vi "Control_giro_v4.vi"() -> ()   [LabVIEW 2025]
uses:
  <vilib>/addons/control/pid/pid.llb/PID (DBL).vi
  <vilib>/addons/control/pid/NI_PID_pid.lvlib
panel:
  in  "Boolean 2":bool
  in  "Boolean":bool
  out "valor_actual_ajustado":dbl
  out "setpoint_ajustado":dbl
  out "PWM":dynamicdata(graph) caption="Square"
  out "Señal B":i16(graph)
  out "Señal A":i16(graph)
  out "output":dbl format="%.2f"
  in  "PID gains":T1={"proportional gain (Kc)"=1.0, "integral time (Ti, min)"=0.01, "derivative time (Td, min)"=0.0} {"derivative time (Td, min)" format="%.3f"; "integral time (Ti, min)" format="%.3f"; "proportional gain (Kc)" format="%.3f"}
  out "Error (°)":dbl
  out "Sensor":dbl(knob) scale=0.0..359.0
  in  "SetPoint":dbl(knob) max=359.0 scale=0.0..359.0
  out "Posición (°)":dbl
  in  "Reestablecer cero":bool
  out "Pulsos":dbl
  in  "stop":bool
  # "ENCODER"
  # "SALIDA"
  # "PID"
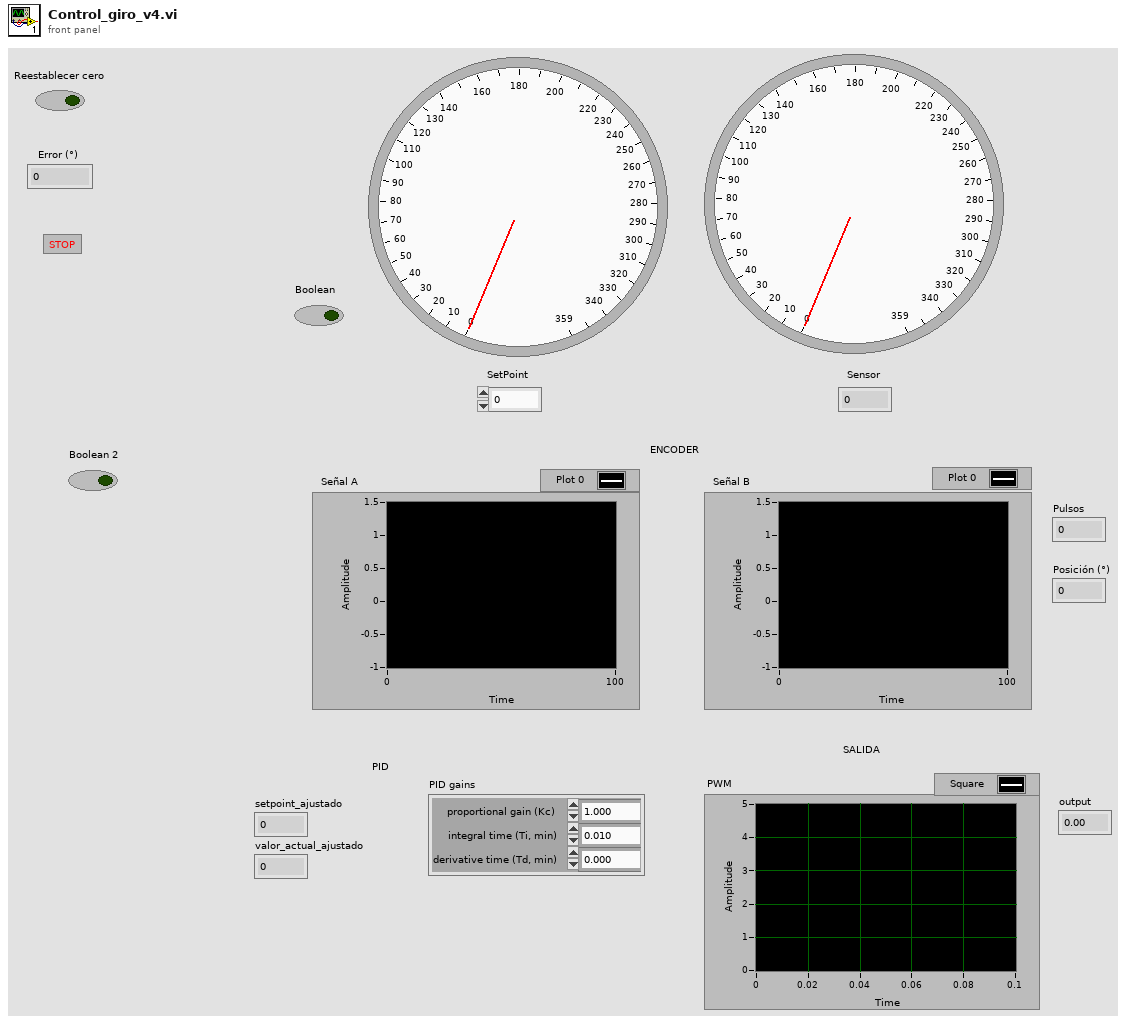
[diagram p1: front panel]
types:
  T1 = cluster{"proportional gain (Kc)":dbl, "integral time (Ti, min)":dbl, "derivative time (Td, min)":dbl}
  T2 = enum16{"Ini", "H1", "H2", "H3", "RES", "A1", "A2", "A3", "SUM"}
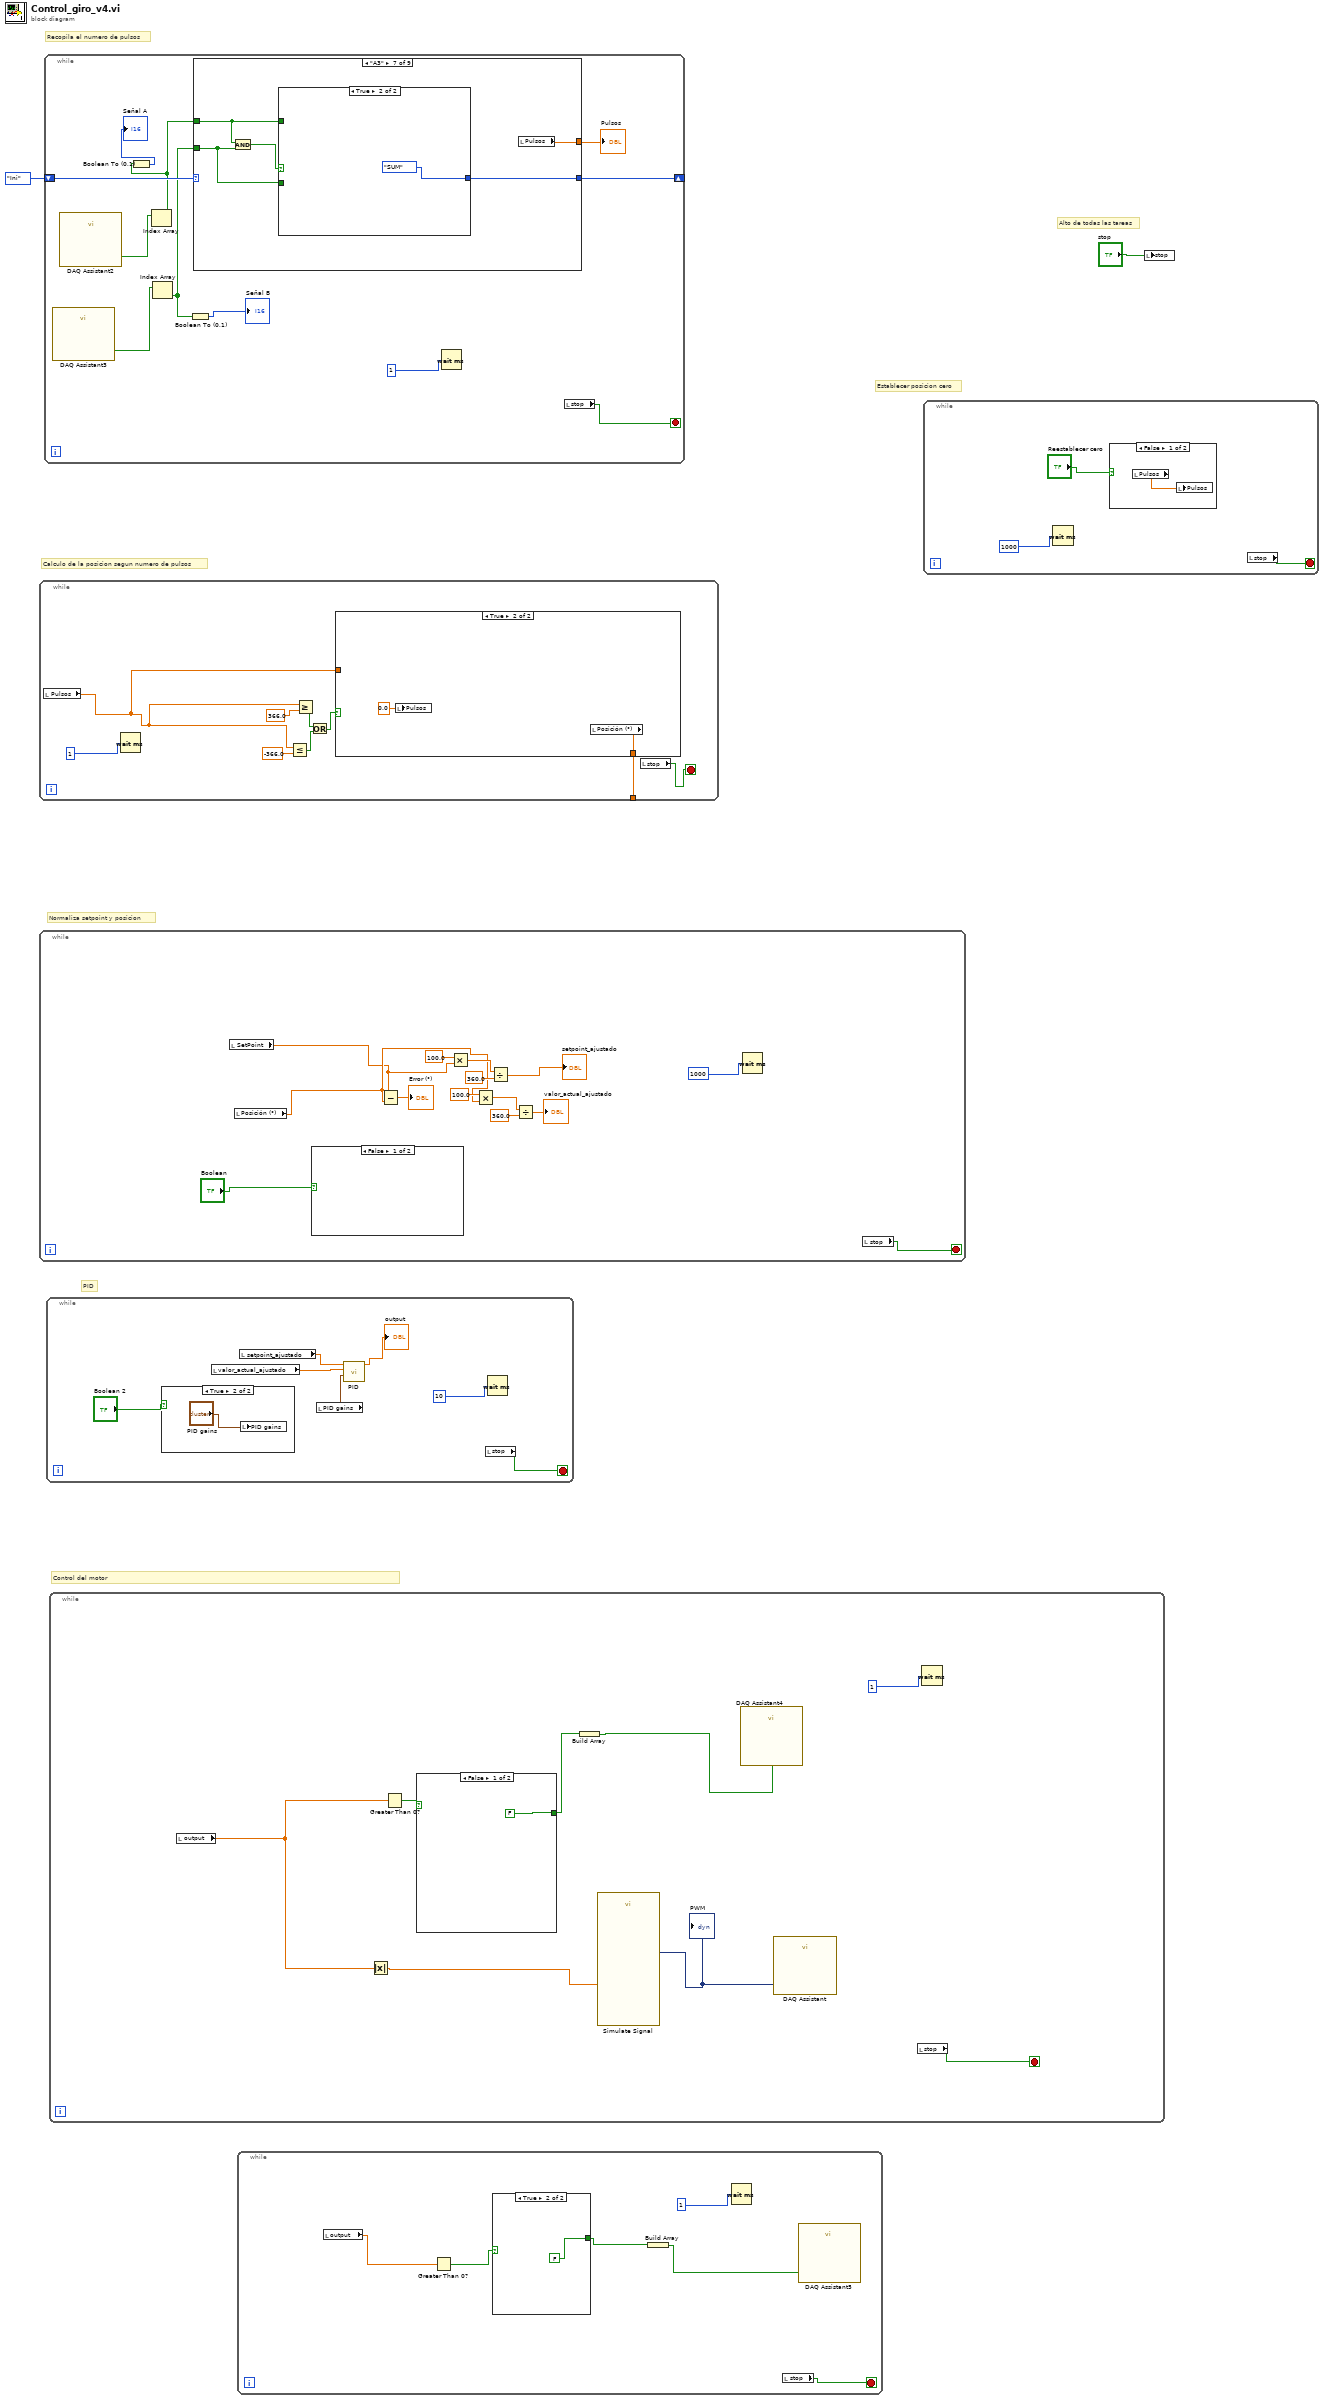
[diagram p0: block diagram]
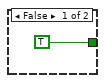
[diagram p2: hidden frame]
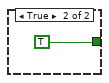
[diagram p4: hidden frame]
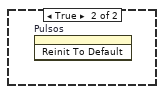
[diagram p5: hidden frame]
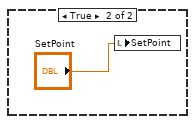
[diagram p6: hidden frame]
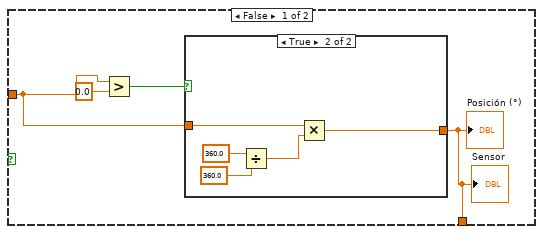
[diagram p7: hidden frame]
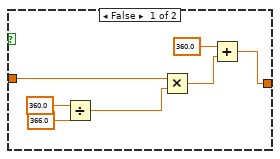
[diagram p8: hidden frame]
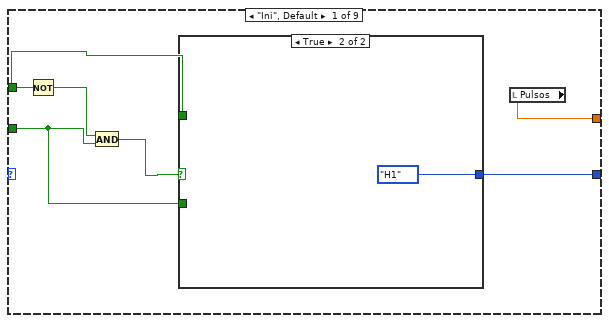
[diagram p9: hidden frame]
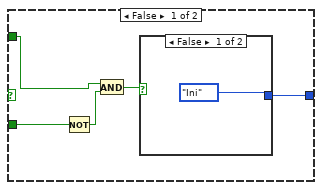
[diagram p10: hidden frame]
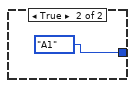
[diagram p11: hidden frame]
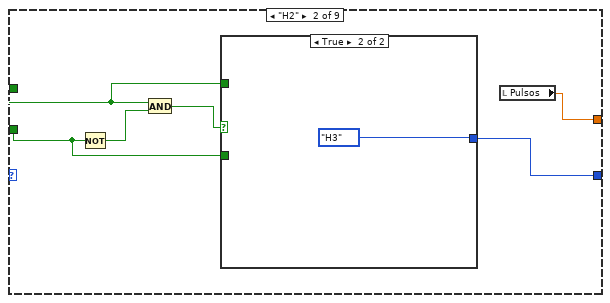
[diagram p12: hidden frame]
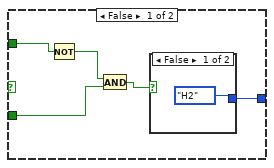
[diagram p13: hidden frame]
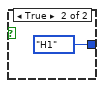
[diagram p14: hidden frame]
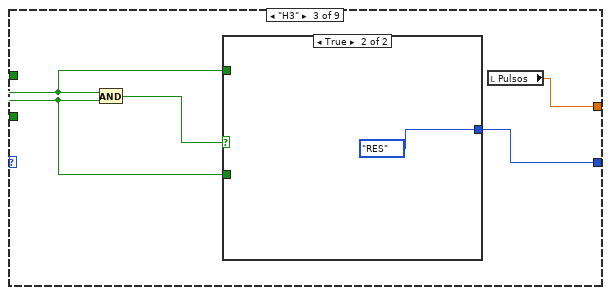
[diagram p15: hidden frame]
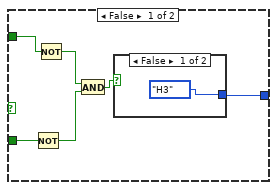
[diagram p16: hidden frame]
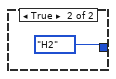
[diagram p17: hidden frame]
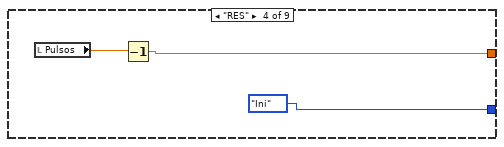
[diagram p18: hidden frame]
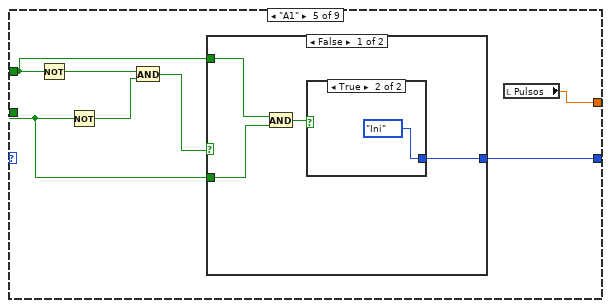
[diagram p19: hidden frame]
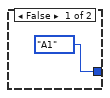
[diagram p20: hidden frame]
diagram:
  # "Establecer posicion cero"
  # "Control del motor"
  # "Calculo de la posicion segun numero de pulsos"
  # "Alto de todas las tareas"
  # "PID"
  # "Normaliza setpoint y posicion"
  # "Recopila el numero de pulsos"
  n1 = while {
    stop <- w9 stop-if-true
    n2 = local read "SetPoint"() -> (w5:dbl)
    n3 = local read "Posición (°)"() -> (w8:dbl)
    n4 = case shown="False" "Boolean" {
      frame False {
      }
      frame True {
        n5 = local write "SetPoint"("SetPoint") -> ()
      }
    }
    n6 = Subtract(x=w5, y=w8) -> (x-y=→"Error (°)":dbl)
    n7 = Multiply(x=100.0, y=w5) -> (x*y=w15:dbl)
    n8 = Multiply(x=100.0, y=w8) -> (x*y=w16:dbl)
    n9 = Divide(x=w15, y=360.0) -> (x/y=→"setpoint_ajustado":dbl)
    n10 = Divide(x=w16, y=360.0) -> (x/y=→"valor_actual_ajustado":dbl)
    n11 = Wait (ms)(milliseconds to wait=1000) -> ()  [unwired: 1 out]
    n12 = local read "stop"() -> (w9:bool)
  }
  n13 = while {
    tunnel: [w21] -> _
    stop <- w20 stop-if-true
    n14 = local read "Pulsos"() -> (w19:dbl)
    n15 = Wait (ms)(milliseconds to wait=1) -> ()  [unwired: 1 out]
    n16 = Less Or Equal?(x=w19, y=-366.0) -> (x <= y?=w25:bool)
    n17 = Greater Or Equal?(x=w19, y=366.0) -> (x >= y?=w24:bool)
    n18 = Or(x=w24, y=w25) -> (x .or. y?=w26:bool)
    n19 = case shown="True" w26 {
      tunnel: w19 -> [w29 _]
      tunnel: [w27 w43] -> w21
      frame False {
        n20 = Greater?(x=w29, y=0.0) -> (0:w28:bool)
        n21 = case shown="True" w28 {
          tunnel: w29 -> [w37 w42]
          tunnel: [w34 w41] -> w27
          frame False {
            n22 = Divide(x=360.0, y=366.0) -> (x/y=w31:dbl)
            n23 = Multiply(x=w37, y=w31) -> (x*y=w35:dbl)
            n24 = Add(x=360.0, y=w35) -> (x+y=w34:dbl)
          }
          frame True {
            n25 = Divide(x=360.0, y=360.0) -> (x/y=w38:dbl)
            n26 = Multiply(x=w42, y=w38) -> (x*y=w41:dbl)
          }
        }
        "Posición (°)" <- w27
        "Sensor" <- w27
      }
      frame True {
        n27 = local write "Pulsos"(0.0 ("Pulsos")) -> ()
        n28 = local read "Posición (°)"() -> (w43:dbl)
      }
    }
    n29 = local read "stop"() -> (w20:bool)
  }
  n30 = while {
    shift-right: [w54] -> _
    shift-left: T2."Ini" -> [w55]
    stop <- w48 stop-if-true
    n31 = call "DAQ Assistant3"() -> ("data"=w47:bool[])  [unwired: 17 in, 2 out]
    n32 = call "DAQ Assistant2"() -> ("data"=w46:bool[])  [unwired: 17 in, 2 out]
    n33 = Index Array(array=w46) -> (element=w50:bool)  [unwired: 1 in]
    n34 = Boolean To (0,1)(Boolean=w50) -> (0, 1=→"Señal A":i16)
    n35 = Index Array(array=w47) -> (element=w53:bool)  [unwired: 1 in]
    n36 = Boolean To (0,1)(Boolean=w53) -> (0, 1=→"Señal B":i16)
    n37 = case shown="\"A3\"" w55 {
      tunnel: w50 -> [w56 w73 w86 _ w103 w118 w130 _ w148]
      tunnel: w53 -> [w59 w72 w85 _ w102 w119 w131 _ w147]
      tunnel: [w60 w71 w87 T2."Ini" w104 w116 w132 T2."Ini" w149] -> w54
      tunnel: [w57 w70 w84 w99 w101 w115 w129 w144 w146] -> w49
      frame "Ini", Default {
        n38 = Not(x=w56) -> (.not. x?=w58:bool)
        n39 = And(x=w58, y=w59) -> (x .and. y?=w61:bool)
        n40 = case shown="True" w61 {
          tunnel: [w62 T2."H1"] -> w60
          tunnel: w59 -> [w66 _]
          tunnel: w56 -> [w65 _]
          frame False {
            n41 = Not(x=w66) -> (.not. x?=w64:bool)
            n42 = And(x=w65, y=w64) -> (x .and. y?=w63:bool)
            n43 = case shown="False" w63 {
              tunnel: [T2."Ini" T2."A1"] -> w62
              frame False {
              }
              frame True {
              }
            }
          }
          frame True {
          }
        }
        n44 = local read "Pulsos"() -> (w57:dbl)
      }
      frame "H2" {
        n45 = Not(x=w72) -> (.not. x?=w75:bool)
        n46 = And(x=w73, y=w75) -> (x .and. y?=w74:bool)
        n47 = case shown="True" w74 {
          tunnel: w73 -> [w80 _]
          tunnel: w72 -> [w79 _]
          tunnel: [w76 T2."H3"] -> w71
          frame False {
            n48 = Not(x=w80) -> (.not. x?=w78:bool)
            n49 = And(x=w78, y=w79) -> (x .and. y?=w77:bool)
            n50 = case shown="False" w77 {
              tunnel: [T2."H2" T2."H1"] -> w76
              frame False {
              }
              frame True {
              }
            }
          }
          frame True {
          }
        }
        n51 = local read "Pulsos"() -> (w70:dbl)
      }
      frame "H3" {
        n52 = And(x=w86, y=w85) -> (x .and. y?=w88:bool)
        n53 = case shown="True" w88 {
          tunnel: [w89 T2."RES"] -> w87
          tunnel: w86 -> [w94 _]
          tunnel: w85 -> [w93 _]
          frame False {
            n54 = Not(x=w93) -> (.not. x?=w90:bool)
            n55 = Not(x=w94) -> (.not. x?=w91:bool)
            n56 = And(x=w91, y=w90) -> (x .and. y?=w92:bool)
            n57 = case shown="False" w92 {
              tunnel: [T2."H3" T2."H2"] -> w89
              frame False {
              }
              frame True {
              }
            }
          }
          frame True {
          }
        }
        n58 = local read "Pulsos"() -> (w84:dbl)
      }
      frame "RES" {
        n59 = local read "Pulsos"() -> (w100:dbl)
        n60 = Decrement(x=w100) -> (x-1=w99:dbl)
      }
      frame "A1" {
        n61 = Not(x=w103) -> (.not. x?=w105:bool)
        n62 = Not(x=w102) -> (.not. x?=w107:bool)
        n63 = And(x=w105, y=w107) -> (x .and. y?=w106:bool)
        n64 = case shown="False" w106 {
          tunnel: [w109 T2."A2"] -> w104
          tunnel: w103 -> [w111 _]
          tunnel: w102 -> [w110 _]
          frame False {
            n65 = And(x=w111, y=w110) -> (x .and. y?=w108:bool)
            n66 = case shown="True" w108 {
              tunnel: [T2."A1" T2."Ini"] -> w109
              frame False {
              }
              frame True {
              }
            }
          }
          frame True {
          }
        }
        n67 = local read "Pulsos"() -> (w101:dbl)
      }
      frame "A2" {
        n68 = Not(x=w118) -> (.not. x?=w121:bool)
        n69 = And(x=w121, y=w119) -> (x .and. y?=w120:bool)
        n70 = Not(x=w119) -> (.not. x?=w117:bool)
        n71 = case shown="False" w120 {
          tunnel: w118 -> [w125 _]
          tunnel: w117 -> [w124 _]
          tunnel: [w122 T2."A3"] -> w116
          frame False {
            n72 = And(x=w125, y=w124) -> (x .and. y?=w123:bool)
            n73 = case shown="True" w123 {
              tunnel: [T2."A2" T2."A1"] -> w122
              frame False {
              }
              frame True {
              }
            }
          }
          frame True {
          }
        }
        n74 = local read "Pulsos"() -> (w115:dbl)
      }
      frame "A3" {
        n75 = And(x=w130, y=w131) -> (x .and. y?=w133:bool)
        n76 = case shown="True" w133 {
          tunnel: [w134 T2."SUM"] -> w132
          tunnel: w131 -> [w139 _]
          tunnel: w130 -> [w138 _]
          frame False {
            n77 = Not(x=w138) -> (.not. x?=w136:bool)
            n78 = Not(x=w139) -> (.not. x?=w135:bool)
            n79 = And(x=w136, y=w135) -> (x .and. y?=w137:bool)
            n80 = case shown="True" w137 {
              tunnel: [T2."A3" T2."A2"] -> w134
              frame False {
              }
              frame True {
              }
            }
          }
          frame True {
          }
        }
        n81 = local read "Pulsos"() -> (w129:dbl)
      }
      frame "SUM" {
        n82 = local read "Pulsos"() -> (w145:dbl)
        n83 = Increment(x=w145) -> (x+1=w144:dbl)
      }
      frame "H1" {
        n84 = Not(x=w147) -> (.not. x?=w151:bool)
        n85 = Not(x=w148) -> (.not. x?=w152:bool)
        n86 = And(x=w152, y=w151) -> (x .and. y?=w150:bool)
        n87 = case shown="False" w150 {
          tunnel: [w154 T2."H2"] -> w149
          tunnel: w148 -> [w156 _]
          tunnel: w147 -> [w155 _]
          frame False {
            n88 = And(x=w156, y=w155) -> (x .and. y?=w153:bool)
            n89 = case shown="True" w153 {
              tunnel: [T2."H1" T2."Ini"] -> w154
              frame False {
              }
              frame True {
              }
            }
          }
          frame True {
          }
        }
        n90 = local read "Pulsos"() -> (w146:dbl)
      }
    }
    "Pulsos" <- w49
    n91 = Wait (ms)(milliseconds to wait=1) -> ()  [unwired: 1 out]
    n92 = local read "stop"() -> (w48:bool)
  }
  n93 = while {
    stop <- w163 stop-if-true
    n94 = case shown="True" "Boolean 2" {
      frame False {
      }
      frame True {
        n95 = local write "PID gains"("PID gains") -> ()
      }
    }
    n96 = local read "valor_actual_ajustado"() -> (w164:dbl)
    n97 = local read "setpoint_ajustado"() -> (w165:dbl)
    n98 = local read "PID gains"() -> (w161:T1)
    n99 = call-poly <vilib>:"PID.vi"("PID gains"=w161, "process variable"=w164, "setpoint"=w165) -> ("output"=→"output":dbl)  [unwired: 7 in, 1 out]
    n100 = local read "stop"() -> (w163:bool)
    n101 = Wait (ms)(milliseconds to wait=10) -> ()  [unwired: 1 out]
  }
  n102 = while {
    stop <- w171 stop-if-true
    n103 = local read "output"() -> (w172:dbl)
    n104 = Absolute Value(x=w172) -> (abs(x)=w174:dbl)
    n105 = Greater Than 0?(x=w172) -> (x > 0?=w175:bool)
    n106 = case shown="False" w175 {
      tunnel: [FALSE TRUE] -> w173
      frame False {
      }
      frame True {
      }
    }
    n107 = Build Array(w173) -> (w169:bool[])
    n108 = call "Simulate Signal"("Duty Cycle (%)"=w174) -> ("Square"=w170:dynamicdata)  [unwired: 13 in, 1 out]
    "PWM" <- w170
    n109 = call "DAQ Assistant4"("data"=w169) -> ()  [unwired: 17 in, 2 out]
    n110 = call "DAQ Assistant"("data"=w170) -> ()  [unwired: 16 in, 3 out]
    n111 = local read "stop"() -> (w171:bool)
    n112 = Wait (ms)(milliseconds to wait=1) -> ()  [unwired: 1 out]
  }
  n113 = while {
    stop <- w183 stop-if-true
    n114 = local read "output"() -> (w182:dbl)
    n115 = Greater Than 0?(x=w182) -> (x > 0?=w181:bool)
    n116 = case shown="True" w181 {
      tunnel: [TRUE FALSE] -> w180
      frame False {
      }
      frame True {
      }
    }
    n117 = Build Array(w180) -> (w179:bool[])
    n118 = Wait (ms)(milliseconds to wait=1) -> ()  [unwired: 1 out]
    n119 = local read "stop"() -> (w183:bool)
    n120 = call "DAQ Assistant5"("data"=w179) -> ()  [unwired: 17 in, 2 out]
  }
  n121 = while {
    stop <- w187 stop-if-true
    n122 = Wait (ms)(milliseconds to wait=1000) -> ()  [unwired: 1 out]
    n123 = case shown="False" "Reestablecer cero" {
      frame False {
        n124 = local read "Pulsos"() -> (w189:dbl)
        n125 = local write "Pulsos"(w189) -> ()
      }
      frame True {
        n126 = invoke on="Pulsos" class="DigNum (strict)" method="Reinit To Default"() -> ()  [unwired: 3 in, 3 out]
      }
    }
    n127 = local read "stop"() -> (w187:bool)
  }
  n128 = local write "stop"("stop") -> ()
